vi "OS_BuildTempFolders.vi"(8 "error in (no error)":errorcluster, 10 "name":string, 11 "path":path) -> (0 "error out":errorcluster, 3 "appended path":path)   [LabVIEW 2024]
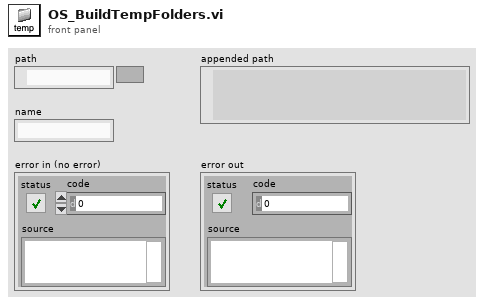
[diagram p1: front panel]
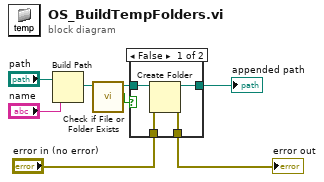
[diagram p0: block diagram]
diagram:
  n1 = Build Path(base path="path", name or relative path="name") -> (appended path=w6:path)
  n2 = call <vilib>:"Check if File or Folder Exists.vi"("path"=w6) -> ("file or folder exists?"=w7:bool)  [unwired: 8 in, 2 out]
  n3 = case shown="False" w7 {
    tunnel: [w11 w12] -> w3
    tunnel: "error in (no error)" -> [w10 w13]
    tunnel: [w9 w13] -> w5
    tunnel: w6 -> [w8 w12]
    frame False {
      n4 = Create Folder(path (use dialog)=w8, error in=w10) -> (created path=w11:path, error out=w9:errorcluster)  [unwired: 1 in, 1 out]
    }
    frame True {
    }
  }
  "error out" <- w5
  "appended path" <- w3
